vi "Waveform_Merge Waveforms.vi"(4 "Size or Time(S)":dbl=1.0, 6 "Size Select":T1(ring), 7 "Digital":bool, 8 "Error":errorcluster, 9 "Waveform To Merge":T2, 10 "Use Merge Dt":bool, 11 "Waveform":T2) -> (0 "Error Out":errorcluster, 2 "Size":i32, 3 "Waveform Out":T2, 5 "Offset Out":i32)   [LabVIEW 2025]
uses:
  Universal Controls/Waveform_Data.ctl
  Universal Controls/Read Write Button.ctl
  <vilib>/Waveform/WDTOps.llb/Check for Equality.vi
  <vilib>/Waveform/WDTOps.llb/Waveform Duration.vi
  <vilib>/Waveform/WDTOps.llb/WDT Waveform Duration DBL.vi
  Dbl Array_Place Line between points.vi
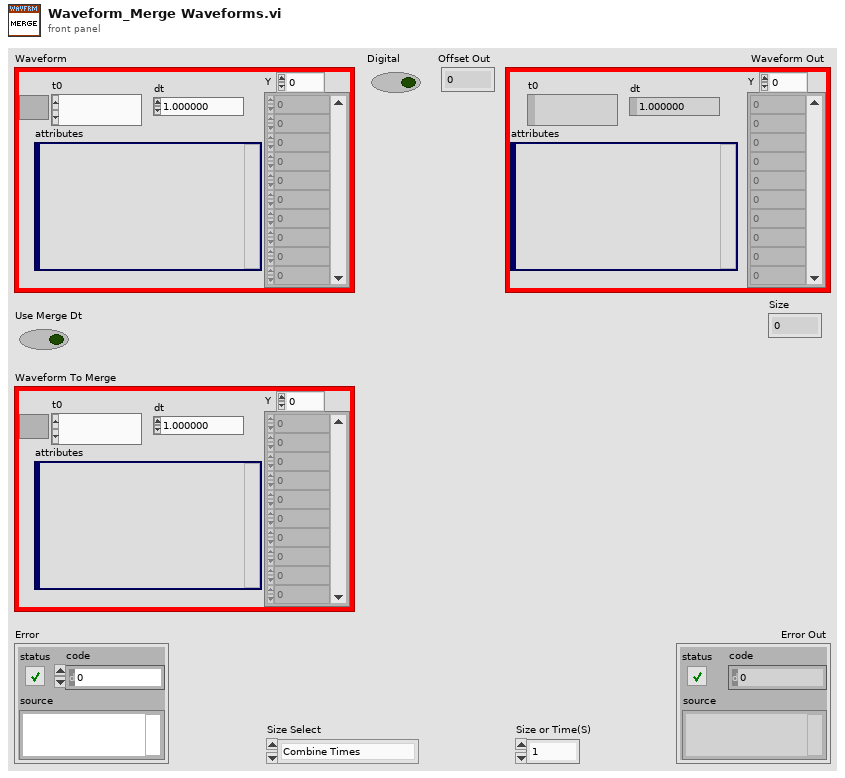
[diagram p1: front panel]
types:
  T1 = enum16{"Combine Times", "Keep Waveform Size", "Set to Size Value", "Set to Time(S) Value"}
  T2 = typedef "Waveform_Data.ctl" = waveform(dbl)
  T3 = typedef "Read Write Button.ctl" = bool
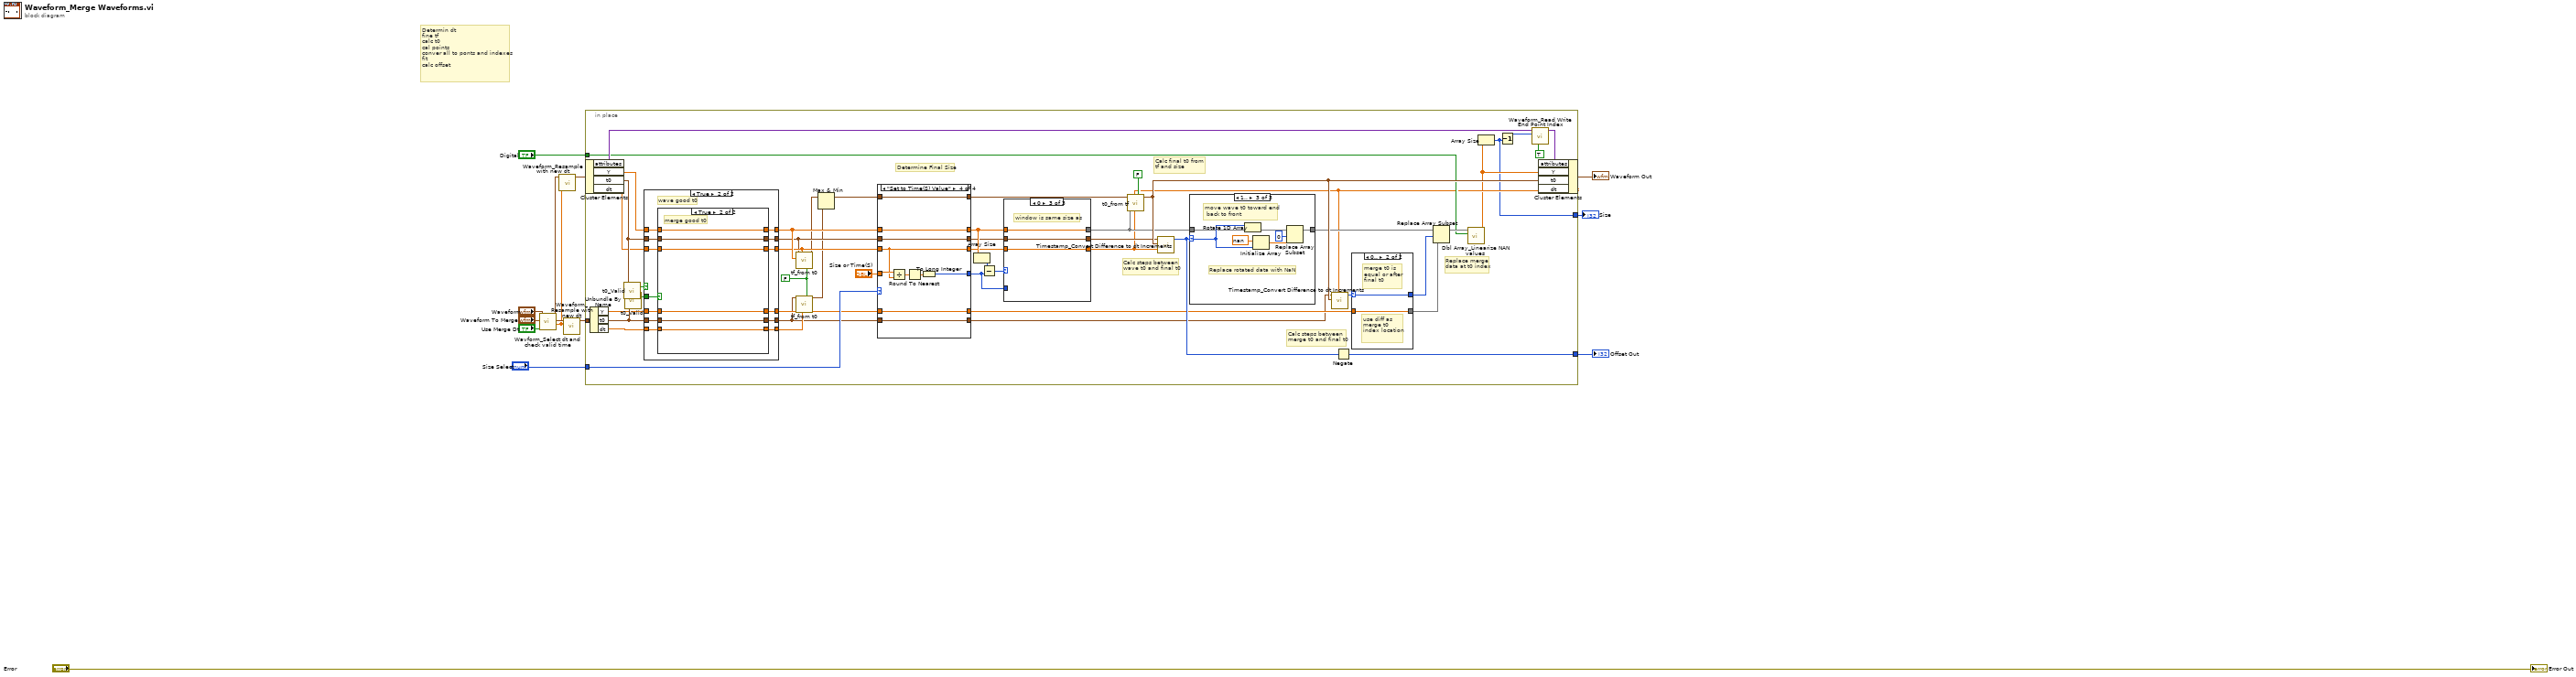
[diagram p0: block diagram]
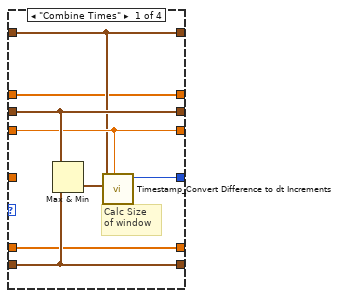
[diagram p2: hidden frame]
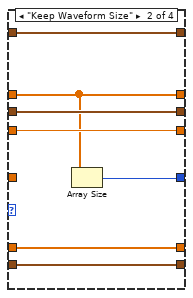
[diagram p3: hidden frame]
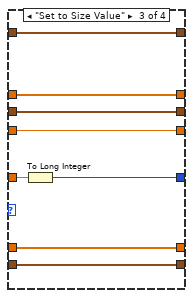
[diagram p4: hidden frame]
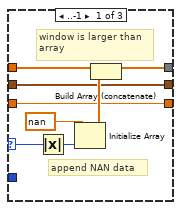
[diagram p5: hidden frame]
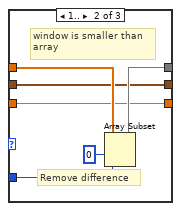
[diagram p6: hidden frame]
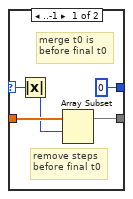
[diagram p7: hidden frame]
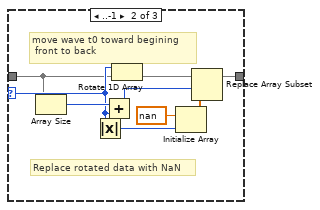
[diagram p9: hidden frame]
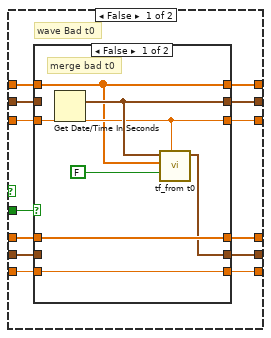
[diagram p10: hidden frame]
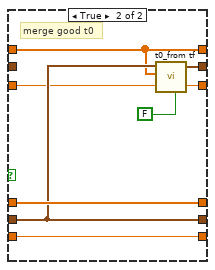
[diagram p11: hidden frame]
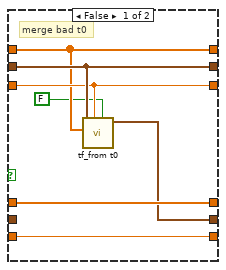
[diagram p12: hidden frame]
diagram:
  # "Determin dt\nfine tf\ncalc t0\ncal points\nconver all to ponts and indexes\nfit\ncalc offset"
  n1 = call "Wavform_Select dt and check valid time.vi"("Use Merge Dt"="Use Merge Dt", "Waveform To Merge"="Waveform To Merge", "Waveform"="Waveform") -> ("Selected Dt Out"=w4:dbl, "Waveform To Merge"=w5:T2, "Waveform"=w6:T2)  [unwired: 6 in]
  n2 = call "Waveform_Resample with new dt.vi"("new dt"=w4, "Waveform to Merge in"=w6) -> ("Waveform to Merge out"=w7:T2)  [unwired: 9 in]
  n3 = call "Waveform_Resample with new dt.vi"("new dt"=w4, "Waveform to Merge in"=w5) -> ("Waveform to Merge out"=w8:T2)  [unwired: 9 in]
  n4 = in-place {
    in-place-border: w8 -> [w63]
    in-place-border: "Size Select" -> [w49]
    in-place-border: "Digital" -> [w42]
    in-place-border: [w41] -> w13
    in-place-border: [w15] -> w1
    w53 = FALSE ("Open(t) Closed(f)")
    # "Determine Final Size"
    # "Calc steps between\nmerge t0 and final t0"
    # "Replace merge\ndata at t0 index"
    # "Calc steps between\nwave t0 and final t0"
    # "Calc final t0 from\ntf and size"
    n5 = in-place-cluster #1(w7) -> ("attributes"=w46:variant, "Y"=w60:dbl[], "t0"=w59:timestamp, "dt"=w58:dbl)
    n6 = Unbundle By Name(w63) -> ("Y"=w55:dbl[], "t0"=w56:timestamp, "dt"=w57:dbl)
    n7 = call "t0_Valid.vi"("T0"=w59) -> ("Valid"=w62:bool)  [unwired: 2 in]
    n8 = call "t0_Valid.vi"("T0"=w56) -> ("Valid"=w61:bool)  [unwired: 2 in]
    n9 = case shown="True" w62 {
      tunnel: w61 -> [w150 w177]
      tunnel: [w149 w176] -> w48
      tunnel: w60 -> [w148 w175]
      tunnel: w59 -> [w147 w174]
      tunnel: w58 -> [w146 w167]
      tunnel: w55 -> [w145 w173]
      tunnel: w56 -> [w144 w172]
      tunnel: w57 -> [w143 w171]
      tunnel: [w142 w170] -> w52
      tunnel: [w141 w169] -> w20
      tunnel: [w140 w168] -> w18
      tunnel: [w139 w166] -> w51
      tunnel: [w138 w165] -> w54
      frame False {
        # "wave Bad t0"
        n10 = case shown="False" w150 {
          tunnel: [w155 w162] -> w149
          tunnel: w148 -> [w153 w159]
          tunnel: w147 -> [_ _]
          tunnel: w146 -> [w154 w158]
          tunnel: w145 -> [w157 w163]
          tunnel: w144 -> [_ w160]
          tunnel: w143 -> [w156 w164]
          tunnel: [w153 w159] -> w142
          tunnel: [w157 w163] -> w141
          tunnel: [w152 w160] -> w140
          tunnel: [w154 w158] -> w139
          tunnel: [w156 w164] -> w138
          frame False {
            # "merge bad t0"
            n11 = Get Date/Time In Seconds() -> (seconds since 1Jan1904=w155:timestamp)
            n12 = call "tf_from t0.vi"("Open(t) Closed(f)"=FALSE ("Open(F) Closed(T)"), "Dt"=w154, "Y"=w153, "T0"=w155) -> ("New Tf Out"=w152:timestamp)  [unwired: 7 in]
          }
          frame True {
            # "merge good t0"
            n13 = call "t0_from tf.vi"("Open(t) Closed(f)"=FALSE ("Open(F) Closed(T)"), "Dt"=w158, "Y"=w159, "Tf"=w160) -> ("New T0 Out"=w162:timestamp)  [unwired: 7 in]
          }
        }
      }
      frame True {
        # "wave good t0"
        n14 = case shown="True" w177 {
          tunnel: [w182 w189] -> w176
          tunnel: w175 -> [w180 w190]
          tunnel: w174 -> [w182 w189]
          tunnel: w167 -> [w181 w186]
          tunnel: w173 -> [w184 w188]
          tunnel: w172 -> [_ w187]
          tunnel: w171 -> [w183 w185]
          tunnel: [w180 w190] -> w170
          tunnel: [w184 w188] -> w169
          tunnel: [w178 w187] -> w168
          tunnel: [w181 w186] -> w166
          tunnel: [w183 w185] -> w165
          frame False {
            # "merge bad t0"
            n15 = call "tf_from t0.vi"("Open(t) Closed(f)"=FALSE, "Dt"=w181, "Y"=w180, "T0"=w182) -> ("New Tf Out"=w178:timestamp)  [unwired: 7 in]
          }
          frame True {
            # "merge good t0"
          }
        }
      }
    }
    n16 = call "tf_from t0.vi"("Open(t) Closed(f)"=w53, "Dt"=w51, "Y"=w52, "T0"=w48) -> ("New Tf Out"=w40:timestamp)  [unwired: 7 in]
    n17 = call "tf_from t0.vi"("Open(t) Closed(f)"=w53, "Dt"=w54, "Y"=w20, "T0"=w18) -> ("New Tf Out"=w39:timestamp)  [unwired: 7 in]
    n18 = Max & Min(x=w40, y=w39) -> (max(x,y)=w30:timestamp)  [unwired: 1 out]
    n19 = case shown="\"Set to Time(S) Value\"" w49 {
      tunnel: w48 -> [w70 w77 w84 w94]
      tunnel: w51 -> [w69 w76 w83 w92]
      tunnel: w18 -> [w68 w72 w79 w87]
      tunnel: w30 -> [w66 w78 w86 w96]
      tunnel: [w67 w74 w81 w89] -> w25
      tunnel: [w66 w78 w86 w96] -> w29
      tunnel: w52 -> [w65 w75 w85 w95]
      tunnel: [w65 w75 w85 w95] -> w24
      tunnel: [w70 w77 w84 w94] -> w23
      tunnel: [w69 w76 w83 w92] -> w22
      tunnel: "Size or Time(S)" -> [_ _ w82 w93]
      tunnel: w20 -> [w64 w73 w80 w88]
      tunnel: [w64 w73 w80 w88] -> w19
      tunnel: [w68 w72 w79 w87] -> w17
      frame "Combine Times" {
        # "Calc Size\nof window"
        n20 = Max & Min(x=w70, y=w68) -> (min(x,y)=w71:timestamp)  [unwired: 1 out]
        n21 = call "Timestamp_Convert Difference to dt Increments.vi"("Dt"=w69, "Start Time"=w71, "End Time"=w66) -> ("Nearest Dt Increment Out"=w67:i32)  [unwired: 6 in, 2 out]
      }
      frame "Keep Waveform Size" {
        n22 = Array Size(array=w75) -> (size(s)=w74:i32)
      }
      frame "Set to Size Value" {
        n23 = To Long Integer(number=w82) -> (32bit integer=w81:i32)
      }
      frame "Set to Time(S) Value" {
        n24 = Divide(x=w93, y=w92) -> (x/y=w91:dbl)
        n25 = Round To Nearest(number=w91) -> (nearest integer value=w90:dbl)
        n26 = To Long Integer(number=w90) -> (32bit integer=w89:i32)
      }
    }
    n27 = Array Size(array=w24) -> (size(s)=w27:i32)
    n28 = Subtract(x=w27, y=w25) -> (x-y=w26:i32)
    n29 = case shown="0" w26 {
      selector: w26 -> [w102 _ _]
      tunnel: w24 -> [w101 w109 w113]
      tunnel: [w100 w108 w113] -> w33
      tunnel: w23 -> [w98 w107 w112]
      tunnel: [w98 w107 w112] -> w31
      tunnel: w22 -> [w97 w106 w111]
      tunnel: [w97 w106 w111] -> w28
      tunnel: w25 -> [_ w105 _]
      frame ..-1 {
        # "append NAN data"
        # "window is larger than\narray"
        n30 = Absolute Value(x=w102) -> (abs(x)=w104:i32)
        n31 = Initialize Array(nan ("element"), w104) -> (w99:dbl[])
        n32 = Build Array (concatenate)(w101, w99) -> (w100:dbl[])
      }
      frame 1.. {
        # "Remove difference"
        # "window is smaller than\narray"
        n33 = Array Subset(array=w109, index=0, length=w105) -> (w108:dbl[])
      }
      frame 0 {
        # "window is same size as"
      }
    }
    n34 = call "t0_from tf.vi"("Open(t) Closed(f)"=FALSE, "Dt"=w28, "Y"=w33, "Tf"=w29) -> ("New T0 Out"=w50:timestamp)  [unwired: 7 in]
    n35 = call "Timestamp_Convert Difference to dt Increments.vi"("Dt"=w28, "Start Time"=w50, "End Time"=w31) -> ("Nearest Dt Increment Out"=w34:i32)  [unwired: 6 in, 2 out]
    n36 = case shown="1.." w34 {
      selector: w34 -> [_ w124 w133]
      tunnel: [w121 w127 w132] -> w38
      tunnel: w33 -> [w121 w122 w131]
      frame 0 {
        # "wave t0 and \nfinal t0 are same"
      }
      frame ..-1 {
        # "Replace rotated data with NaN"
        # "move wave t0 toward begining\n front to back"
        n37 = Array Size(array=w122) -> (size(s)=w125:i32)
        n38 = Absolute Value(x=w124) -> (abs(x)=w129:i32)
        n39 = Add(x=w125, y=w124) -> (x+y=w123:i32)
        n40 = Rotate 1D Array(1:w122, 2:w124) -> (0:w128:dbl[])
        n41 = Initialize Array(nan ("element"), w129) -> (w126:dbl[])
        n42 = Replace Array Subset(array=w128, new element=w126, index=w123) -> (w127:dbl[])
      }
      frame 1.. {
        # "Replace rotated data with NaN"
        # "move wave t0 toward end\n back to front"
        n43 = Rotate 1D Array(1:w131, 2:w133) -> (0:w136:dbl[])
        n44 = Initialize Array(nan ("element"), w133) -> (w135:dbl[])
        n45 = Replace Array Subset(array=w136, new element=w135, index=0) -> (w132:dbl[])
      }
    }
    n46 = call "Timestamp_Convert Difference to dt Increments.vi"("Dt"=w28, "Start Time"=w50, "End Time"=w17) -> ("Nearest Dt Increment Out"=w37:i32)  [unwired: 6 in, 2 out]
    n47 = Negate(x=w34) -> (-x=w41:i32)
    n48 = case shown="0.." w37 {
      selector: w37 -> [w115 w119]
      tunnel: w19 -> [w117 w120]
      tunnel: [w116 w120] -> w36
      tunnel: [0 ("Nearest Dt Increment Out") w119] -> w35
      frame ..-1 {
        # "remove steps\nbefore final t0"
        # "merge t0 is\nbefore final t0"
        n49 = Absolute Value(x=w115) -> (abs(x)=w114:i32)
        n50 = Array Subset(array=w117, index=w114) -> (w116:dbl[])  [unwired: 1 in]
      }
      frame 0.. {
        # "use diff as merge t0\nindex location"
        # "merge t0 is\nequal or after\nfinal t0"
      }
    }
    n51 = Replace Array Subset(array=w38, new element=w36, index=w35) -> (w43:dbl[])
    n52 = call "Dbl Array_Linearize NAN values.vi"("Digital"=w42, "Dbl Array"=w43) -> ("Dbl Array Out"=w16:dbl[])  [unwired: 8 in, 1 out]
    n53 = Array Size(array=w16) -> (size(s)=w15:i32)
    n54 = Decrement(x=w15) -> (x-1=w44:i32)
    n55 = call "Waveform_Read Write End Point Index.vi"("Read(f)\nWrite(t)"=T3 TRUE ("Read(f)\nWrite(t)"), "End Point"=w44, "Waveform Attributes"=w46) -> ("Waveform Attributes Out"=w45:variant)  [unwired: 5 in, 3 out]
    n56 = in-place-cluster #1("attributes"=w45, "Y"=w16, "t0"=w50, "dt"=w28) -> (→"Waveform Out":T2)
  }
  "Offset Out" <- w13
  "Size" <- w1
  "Error Out" <- "Error"
